vi "filtering outliers.vi"() -> ()   [LabVIEW 2015]
uses:
  <vilib>/Utility/file.llb/Read Delimited Spreadsheet (string).vi
  <vilib>/Utility/file.llb/Write Delimited Spreadsheet (string).vi
  <vilib>/express/express arith-compare/Formula/XNode/ExpressFormulaBlockNode.xnode
  <vilib>/Analysis/NI_AALBase.lvlib
panel:
  out "all rows":string[][](array[string])
  out "列":i32
  out "盆数":i32
  out "all rows 2":string[][](array[string])
  in  "error in (no error)":errorcluster
  out "当前txt":string
  in  "file path (dialog if empty)":path=path "H:/fh/传输D/2017 油菜/张国方-表型平台油菜数据整理-2018-3-5/张国方-油菜盐胁迫高光谱-2018-3-6/高光谱第二次-CK.txt"
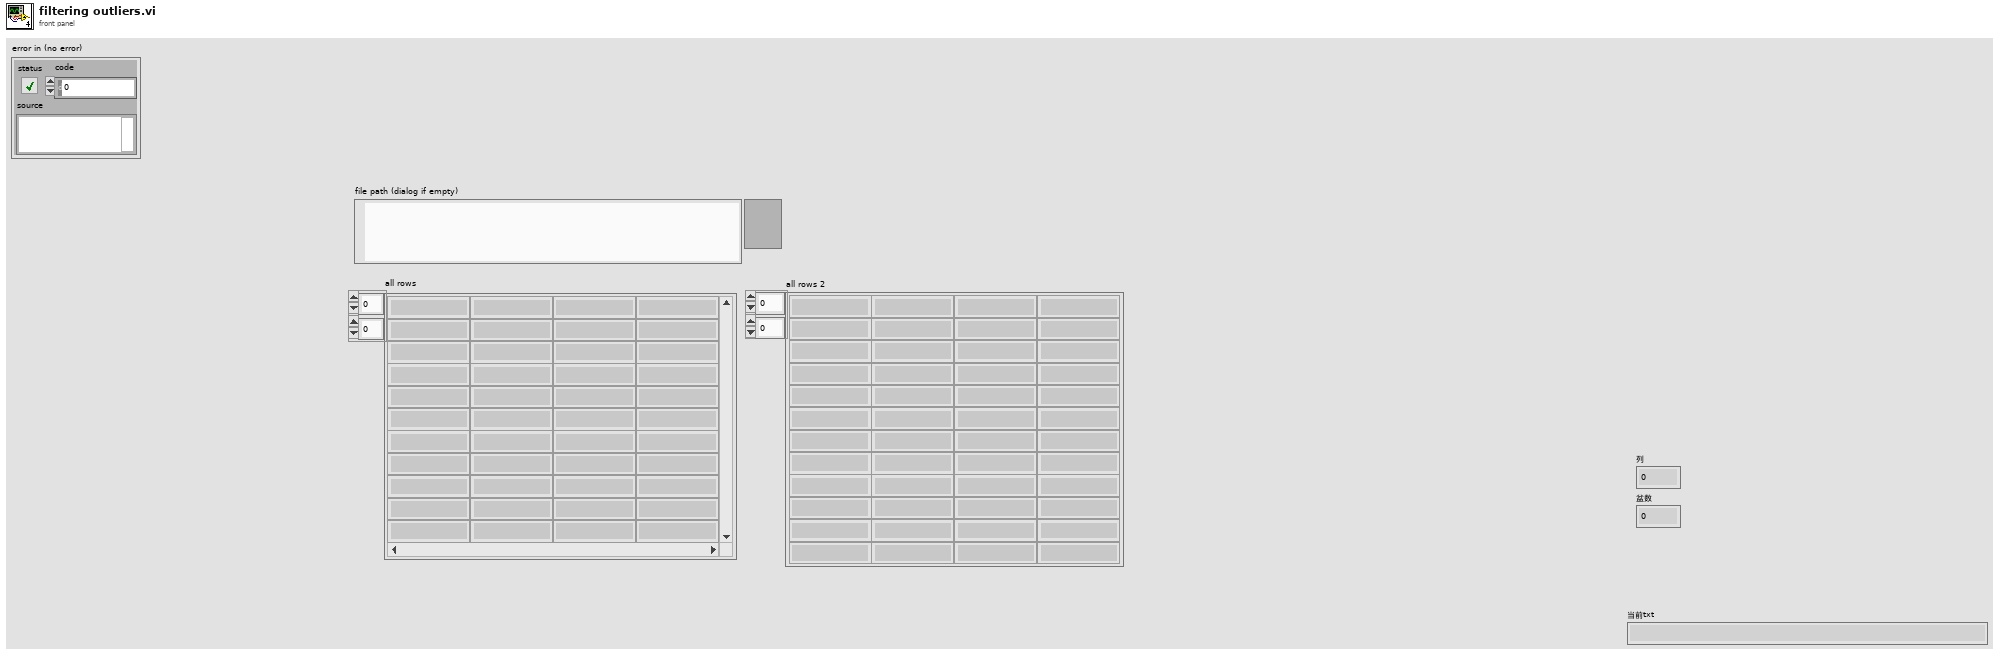
[diagram p1: front panel]
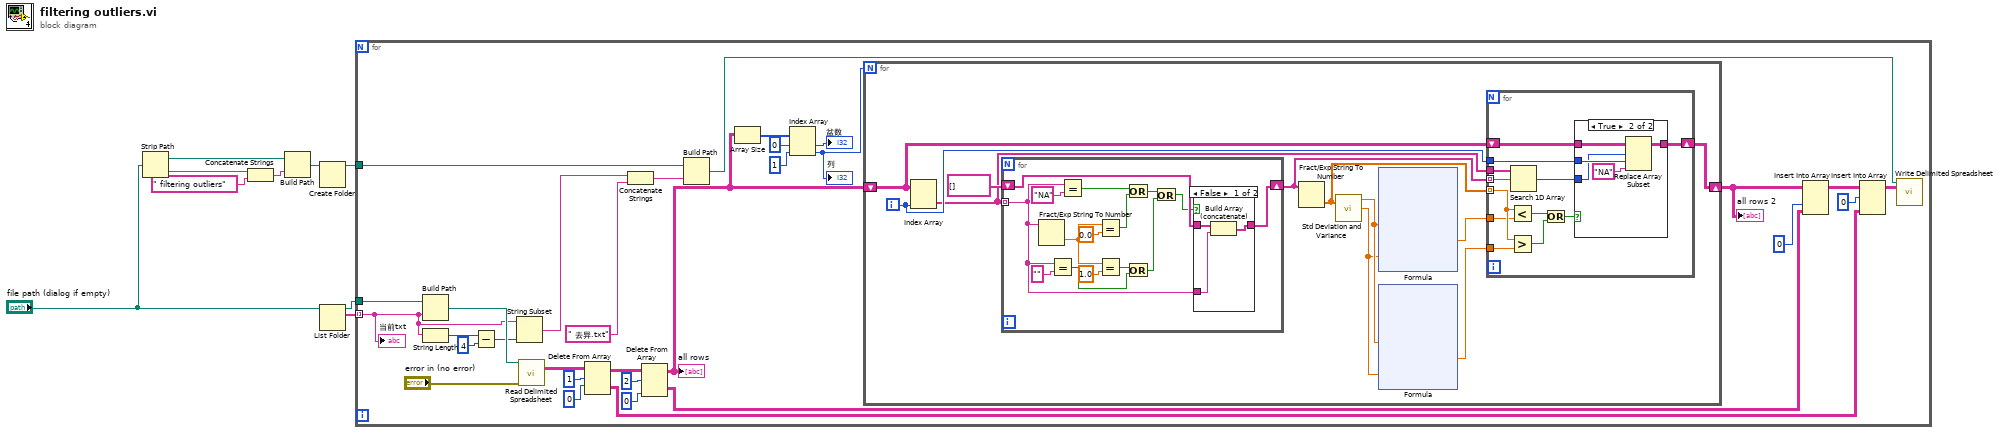
[diagram p0: block diagram]
diagram:
  n1 = Strip Path(path="file path (dialog if empty)") -> (stripped path=w4:path, name=w6:string)
  n2 = Concatenate Strings(w6, " filtering outliers" ("string")) -> (w3:string)
  n3 = Build Path(base path=w4, name or relative path=w3) -> (appended path=w2:path)
  n4 = Create Folder(path (use dialog)=w2) -> (created path=w1:path)  [unwired: 2 in, 2 out]
  n5 = List Folder(path="file path (dialog if empty)") -> (path out=w9:path, filenames=w8:string[])  [unwired: 3 in, 2 out]
  n6 = for {
    tunnel: w9 -> [w27]
    tunnel: w8 -> [w25] mode=indexing
    tunnel: w1 -> [w19]
    n7 = Build Path(base path=w27, name or relative path=w25) -> (appended path=w26:path)
    n8 = String Length(string=w25) -> (length=w24:i32)
    n9 = Subtract(x=w24, y=4) -> (x-y=w22:i32)
    n10 = String Subset(string=w25, length (rest)=w22) -> (substring=w21:string)  [unwired: 1 in]
    n11 = call-poly <vilib>:"Read Delimited Spreadsheet.vi"("file path (dialog if empty)"=w26, "error in (no error)"="error in (no error)") -> ("all rows"=w40:string[][])  [unwired: 8 in, 5 out]
    n12 = Delete From Array(array=w40, length=1, index (row)=0) -> (deleted portion=w28:string[][], array with subset deleted=w37:string[][])  [unwired: 1 in]
    n13 = Concatenate Strings(w21, " 去异.txt" ("string")) -> (w18:string)
    n14 = Delete From Array(array=w37, length=2, index (col)=0 ("disabled index (col)")) -> (deleted portion=w29:string[][], array with subset deleted=w30:string[][])  [unwired: 1 in]
    "all rows" <- w30
    n15 = Build Path(base path=w19, name or relative path=w18) -> (appended path=w17:path)
    n16 = Array Size(array=w30) -> (size(s)=w34:i32[])
    n17 = Index Array(array=w34, index #1=0 ("index"), index #2=1 ("index")) -> (element #1=→"盆数":i32, element #2=w10:i32)
    "列" <- w10
    n18 = for {
      N: w10 -> [_]
      shift-right: [w44] -> w16
      shift-left: w30 -> [w46]
      i -> [w45]
      n19 = Index Array(array=w46, index (col)=w45) -> (element=w42:string[])  [unwired: 1 in]
      n20 = for {
        tunnel: w42 -> [w58] mode=indexing
        shift-right: [w64] -> w41
        shift-left: string[] [] ("subarray") -> [w65]
        n21 = Fract/Exp String To Number(string=w58) -> (number=w60:dbl)  [unwired: 3 in, 1 out]
        n22 = Equal?(x=w58, y="") -> (x = y?=w55:bool)
        n23 = Equal?(x=w58, y="NA") -> (x = y?=w62:bool)
        n24 = Equal?(x=w60, y=0.0) -> (x = y?=w61:bool)
        n25 = Equal?(x=w60, y=1.0) -> (x = y?=w56:bool)
        n26 = Or(x=w62, y=w61) -> (x .or. y?=w54:bool)
        n27 = Or(x=w56, y=w55) -> (x .or. y?=w53:bool)
        n28 = Or(x=w54, y=w53) -> (x .or. y?=w52:bool)
        n29 = case shown="False" w52 {
          tunnel: w65 -> [w69 w70]
          tunnel: w58 -> [w68 _]
          tunnel: [w67 w70] -> w64
          frame False {
            n30 = Build Array (concatenate)(w69, w68) -> (w67:string[])
          }
          frame True {
          }
        }
      }
      n31 = Fract/Exp String To Number(string=w41) -> (number=w49:dbl[])  [unwired: 3 in, 1 out]
      n32 = call <vilib>:"Std Deviation and Variance.vi"("X"=w49) -> ("mean"=w51:dbl, "standard deviation"=w50:dbl)  [unwired: 1 in, 1 out]
      n33 = xnode "Formula"("mean"=w51, "s"=w50) -> ("Result"=w48:dbl)  [unwired: 1 in, 1 out]
      n34 = xnode "Formula"("mean"=w51, "s"=w50) -> ("Result"=w47:dbl)  [unwired: 1 in, 1 out]
      n35 = for {
        tunnel: w49 -> [w82] mode=indexing
        tunnel: w48 -> [w81]
        tunnel: w47 -> [w80]
        shift-right: [w74] -> w44
        shift-left: w46 -> [w76]
        tunnel: w45 -> [w75]
        tunnel: w42 -> [w73]
        tunnel: w41 -> [w72] mode=indexing
        n36 = Less?(x=w82, y=w81) -> (x < y?=w79:bool)
        n37 = Greater?(x=w82, y=w80) -> (0:w78:bool)
        n38 = Search 1D Array(1D array=w73, element=w72) -> (index of element=w71:i32)  [unwired: 1 in]
        n39 = Or(x=w79, y=w78) -> (x .or. y?=w77:bool)
        n40 = case shown="True" w77 {
          tunnel: w76 -> [w83 w88]
          tunnel: w75 -> [_ w87]
          tunnel: [w83 w85] -> w74
          tunnel: w71 -> [_ w84]
          frame False {
          }
          frame True {
            n41 = Replace Array Subset(array=w88, new element="NA" ("new element/subarray"), index (row)=w84, index (col)=w87) -> (w85:string[][])
          }
        }
      }
    }
    "all rows 2" <- w16
    n42 = Insert Into Array(array=w16, index (col)=0 ("disabled index (col)"), new element=w29) -> (w14:string[][])  [unwired: 1 in]
    n43 = Insert Into Array(array=w14, index (row)=0, new element=w28) -> (w12:string[][])  [unwired: 1 in]
    n44 = call-poly <vilib>:"Write Delimited Spreadsheet.vi"("file path (dialog if empty)"=w17, "2D data"=w12) -> ()  [unwired: 12 in, 2 out]
    "当前txt" <- w25
  }
